vi "PDW gen.vi"() -> ()   [LabVIEW 2021]
uses:
  emitter params.ctl
  pdw.ctl
  <vilib>/numeric/Random Number (Range) DBL.vi
  <vilib>/numeric/Random Number (Range) U64.vi
  <vilib>/numeric/sub_Random U32.vi
panel:
  out "lfm lost":bool
  in  "Tab Control":T1(tab)
  in  "end time (sec)":dbl=50.0
  in  "start time (sec)":dbl format="%#_13g"
  in  "Fs":i32=200000000 format="%.0p"
  in  "tdms output file path":path=path "C:/Users/NI/Documents/chaim/chaim__Tx/data/pulses.tdms"
  in  "center frequency (Hz)":dbl=2000000000.0 format="%#_13p"
  in  "amp range":cluster{dbl, dbl}(slide)={-21.121351766513058, -25.88325652841782} scale=0.0..-50.0 scale format="%#_g dB"
  in  "span range":cluster{dbl, dbl}(slide)={1634128.9560392164, 2964508.639841233} scale=1000000.0..30000000.0 scale format="%#_6p Hz"
  in  "hop rate range":cluster{dbl, dbl}(slide)={2.0915680786684536, 3.1385684721559217} scale=1.0..3000.0 scale format="%#_6p"
  in  "D.C range":cluster{dbl, dbl}(slide)={0.5407066052227343, 0.5038402457757296} scale=0.0..1.0
  in  "f band range":cluster{dbl, dbl}(slide)={-77296466.97388633, 78525345.62211981} scale=-80000000.0..80000000.0 scale format="%#_6p Hz"
  in  "CW":bool=TRUE
  in  "LFM":bool=TRUE
  in  "BPSK":bool=TRUE
  in  "QPSK":bool=TRUE
  in  "num of frequncyes":cluster{i32, i32}(slide)={2, 1} scale=1.0..300.0
  in  "num of hoopers":i32(slide)=10 scale=0.0..16.0
  in  "modulation depth":cluster{dbl, dbl}(slide)={67532.40039072247, 205475.5312375231} scale=10000.0..3000000.0 scale format="%#_6p Hz"
  in  "user bulid emmiters":T2[](array[typedef]) {"mod depth" format="%.0p"; "f set" format="%#_6p"}
  out "PDW":T3={"PW"=44197525, "frequency shift"=-0.34743934348748695, "amp"=0.06598663330078125, "mode type"=4, "mode depth"=1109, "mode filter"=0}
  out "saturation":bool
  out "num of pulses":i32=1261
  # "available modulations:"
  # "mode type:\n0-CW\n3-LFM\n4-BPSK\n5-QPSK"
  # "mode type:\n0-CW\n3-LFM\n4-BPSK\n5-QPSK"
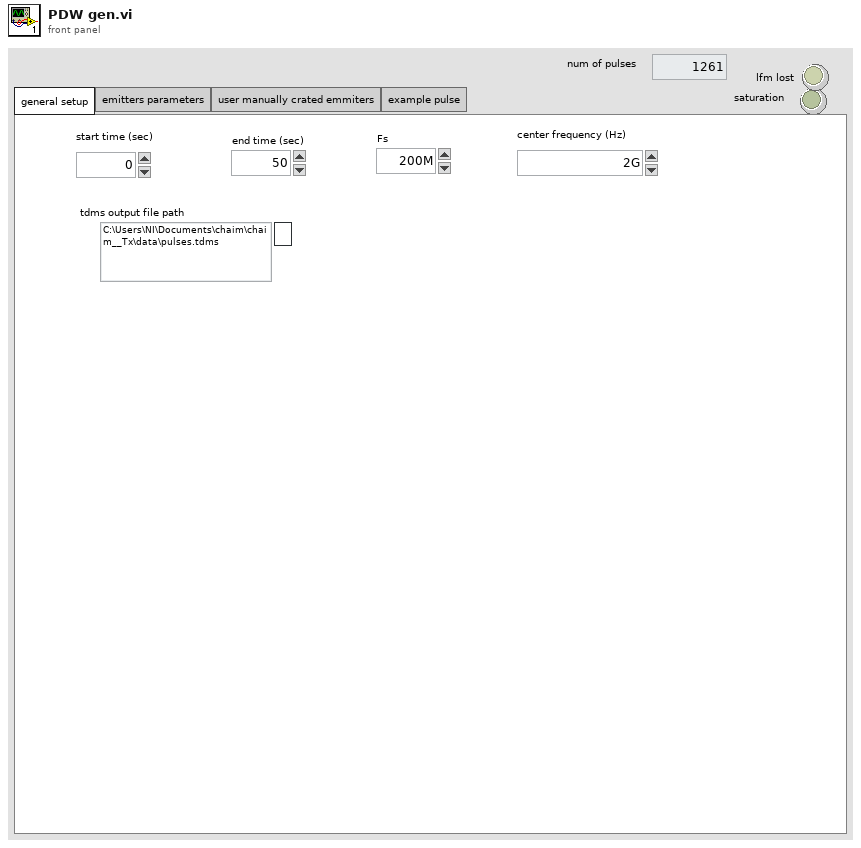
[diagram p1: front panel]
types:
  T1 = enum32{"general setup", "emitters parameters", "user manually crated emmiters", "example pulse"}
  T2 = typedef "emitter params.ctl" = cluster{"f set":dbl[], "hop rate (Hz)":dbl, "d.c.":dbl, "amp (dB)":dbl, "mod type":u8, "mod depth":dbl}
  T3 = typedef "pdw.ctl" = cluster{"PW":u32, "frequency shift":fxp<+/-,48,0>, "amp":fxp<+/-,18,1>, "mode type":u8, "mode depth":u32, "mode filter":u8}
  T4 = enum16{"open", "open or create", "create or replace", "create", "open (read-only)"}
  T5 = cluster{"start time":dbl, "Numeric":dbl, dbl, "amp (dB)":dbl, "mod type":u8, "mod file 2":u8, "mod depth":dbl, "pulse filter":u16, "mod filter 2":u16}[]
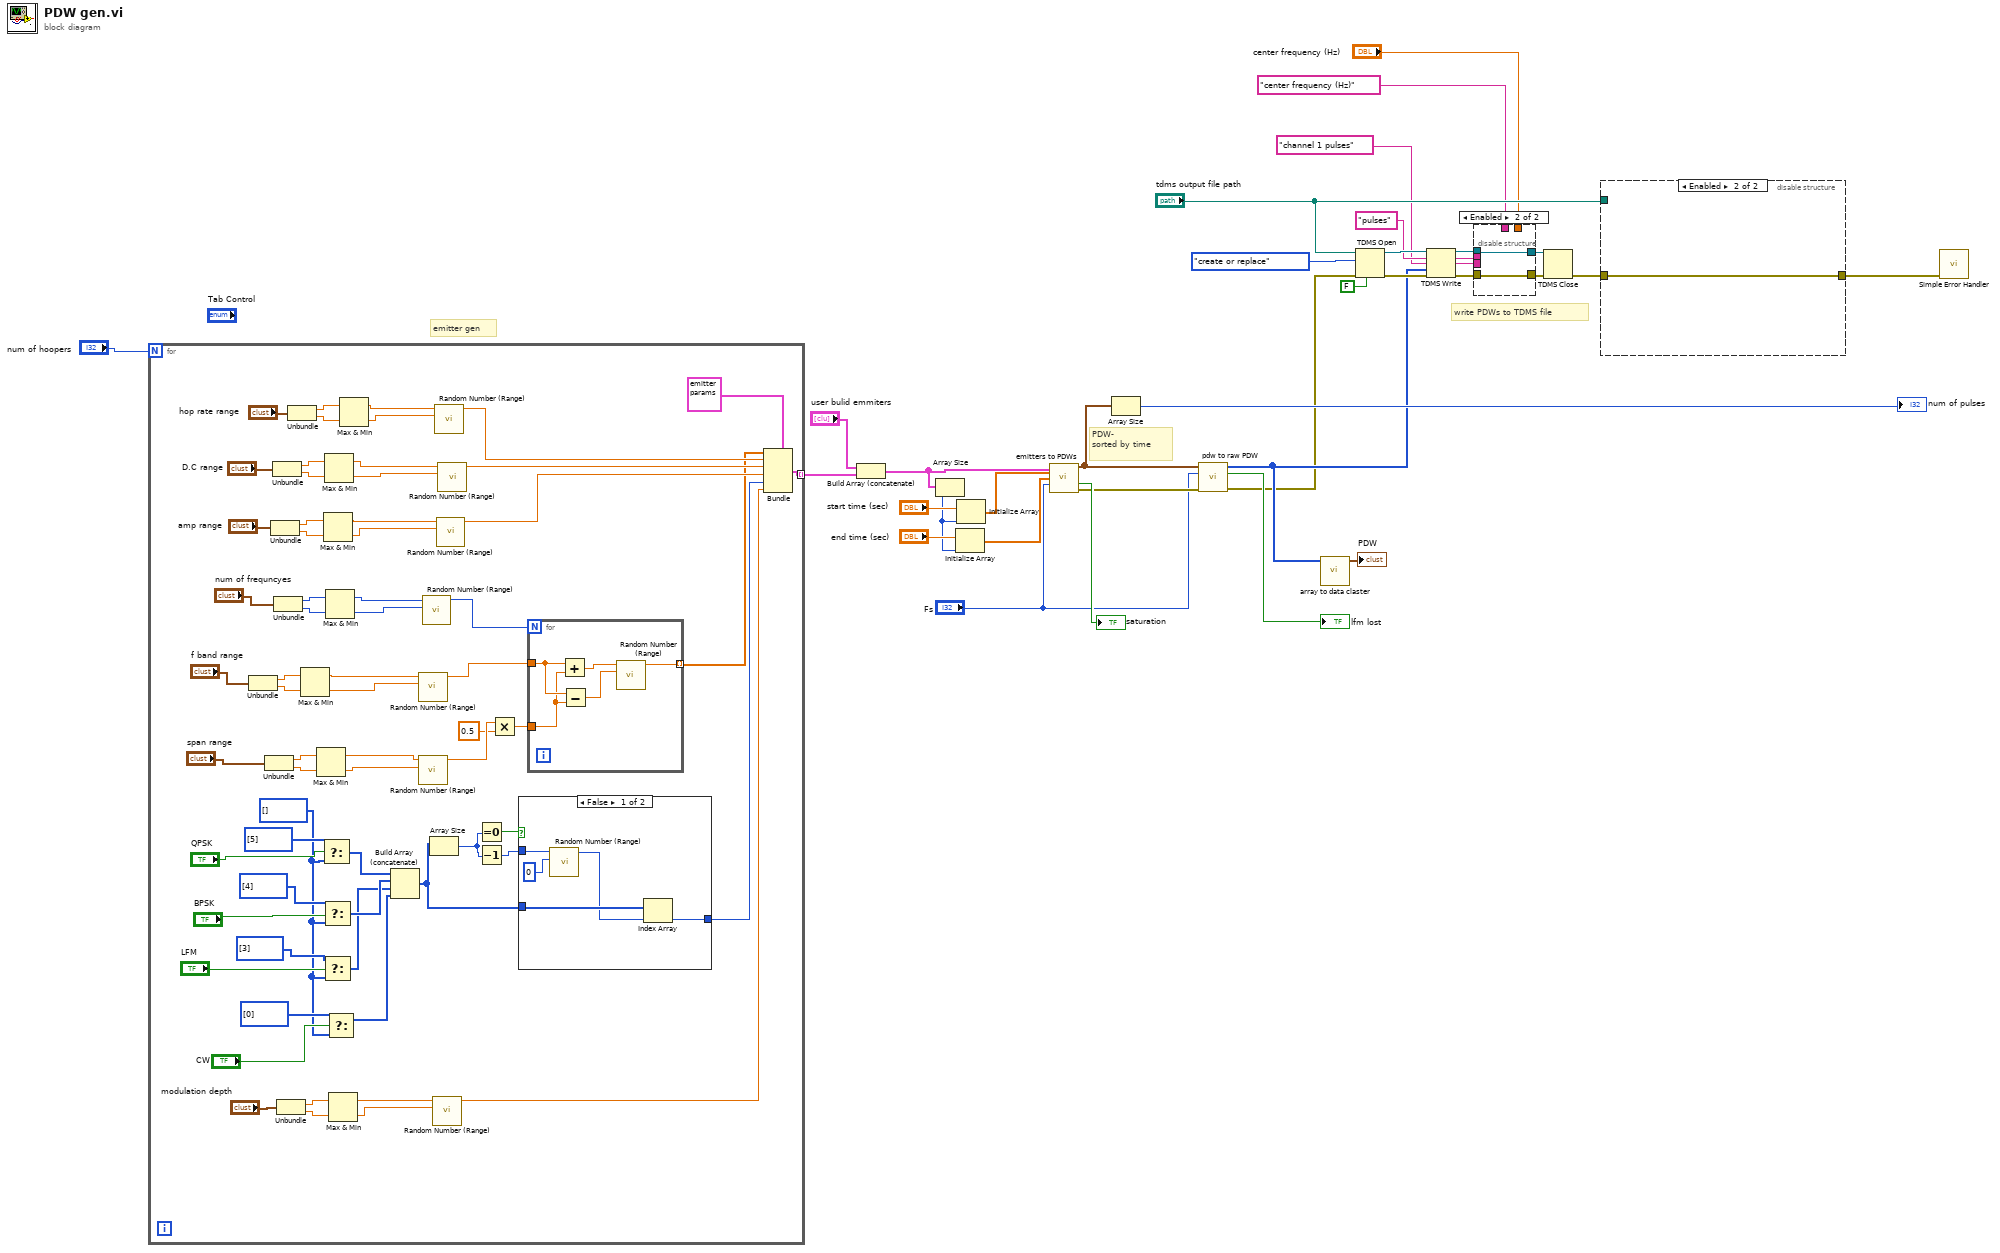
[diagram p0: block diagram]
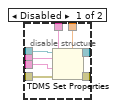
[diagram p2: hidden frame]
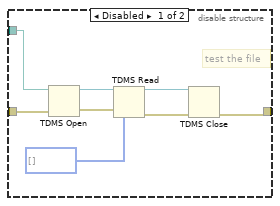
[diagram p3: hidden frame]
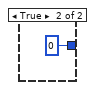
[diagram p4: hidden frame]
diagram:
  # "write PDWs to TDMS file"
  # "PDW- \nsorted by time"
  # "emitter gen"
  n1 = for {
    N: "num of hoopers" -> [_]
    tunnel: [w91] -> w34 mode=indexing
    w36 = u8[] []
    n2 = Unbundle("f band range") -> (w69:dbl, w68:dbl)
    n3 = Unbundle("span range") -> (w63:dbl, w64:dbl)
    n4 = Unbundle("amp range") -> (w87:dbl, w86:dbl)
    n5 = Unbundle("D.C range") -> (w83:dbl, w84:dbl)
    n6 = Unbundle("num of frequncyes") -> (w73:i32, w74:i32)
    n7 = Unbundle("modulation depth") -> (w59:dbl, w58:dbl)
    n8 = Unbundle("hop rate range") -> (w79:dbl, w78:dbl)
    n9 = Max & Min(x=w69, y=w68) -> (max(x,y)=w66:dbl, min(x,y)=w65:dbl)
    n10 = Max & Min(x=w63, y=w64) -> (max(x,y)=w62:dbl, min(x,y)=w61:dbl)
    n11 = Select(t=u8[] [5], s="QPSK", f=w36) -> (s? t:f=w50:u8[])
    n12 = Max & Min(x=w87, y=w86) -> (max(x,y)=w89:dbl, min(x,y)=w88:dbl)
    n13 = Select(t=u8[] [4], s="BPSK", f=w36) -> (s? t:f=w49:u8[])
    n14 = Select(t=u8[] [3], s="LFM", f=w36) -> (s? t:f=w48:u8[])
    n15 = Max & Min(x=w83, y=w84) -> (max(x,y)=w82:dbl, min(x,y)=w81:dbl)
    n16 = Max & Min(x=w73, y=w74) -> (max(x,y)=w71:i32, min(x,y)=w70:i32)
    n17 = Select(t=u8[] [0], s="CW", f=w36) -> (s? t:f=w47:u8[])
    n18 = Max & Min(x=w59, y=w58) -> (max(x,y)=w56:dbl, min(x,y)=w55:dbl)
    n19 = Max & Min(x=w79, y=w78) -> (max(x,y)=w76:dbl, min(x,y)=w75:dbl)
    n20 = Build Array (concatenate)(w50, w49, w48, w47) -> (w46:u8[])
    n21 = call-poly <vilib>:"Random Number (Range).vi"("lower bound (0)"=w65, "upper bound (100)"=w66) -> ("number"=w94:dbl)  [unwired: 9 in]
    n22 = call-poly <vilib>:"Random Number (Range).vi"("lower bound (0)"=w61, "upper bound (100)"=w62) -> ("number"=w96:dbl)  [unwired: 9 in]
    n23 = call-poly <vilib>:"Random Number (Range).vi"("lower bound (0)"=w70, "upper bound (100)"=w71) -> ("number"=w90:u64)  [unwired: 9 in]
    n24 = Array Size(array=w46) -> (size(s)=w42:i32)
    n25 = call-poly <vilib>:"Random Number (Range).vi"("lower bound (0)"=w55, "upper bound (100)"=w56) -> ("number"=w43:dbl)  [unwired: 9 in]
    n26 = call-poly <vilib>:"Random Number (Range).vi"("lower bound (0)"=w75, "upper bound (100)"=w76) -> ("number"=w99:dbl)  [unwired: 9 in]
    n27 = call-poly <vilib>:"Random Number (Range).vi"("lower bound (0)"=w88, "upper bound (100)"=w89) -> ("number"=w97:dbl)  [unwired: 9 in]
    n28 = call-poly <vilib>:"Random Number (Range).vi"("lower bound (0)"=w81, "upper bound (100)"=w82) -> ("number"=w98:dbl)  [unwired: 9 in]
    n29 = Equal To 0?(x=w42) -> (x = 0?=w44:bool)
    n30 = Decrement(x=w42) -> (x-1=w41:i32)
    n31 = Multiply(x=w96, y=0.5) -> (x*y=w93:dbl)
    n32 = case shown="False" w44 {
      tunnel: w46 -> [w104 _]
      tunnel: [w102 u8 0 ("unsigned 8bit integer")] -> w45
      tunnel: w41 -> [w101 _]
      frame False {
        n33 = call-poly <vilib>:"Random Number (Range).vi"("lower bound (0)"=u64 0, "upper bound (100)"=w101) -> ("number"=w103:u64)  [unwired: 9 in]
        n34 = Index Array(array=w104, index=w103) -> (element=w102:u8)
      }
      frame True {
      }
    }
    n35 = for {
      N: w90 -> [_]
      tunnel: w94 -> [w111]
      tunnel: w93 -> [w110]
      tunnel: [w107] -> w92 mode=indexing
      n36 = Add(x=w111, y=w110) -> (x+y=w108:dbl)
      n37 = Subtract(x=w111, y=w110) -> (x-y=w109:dbl)
      n38 = call-poly <vilib>:"Random Number (Range).vi"("lower bound (0)"=w109, "upper bound (100)"=w108) -> ("number"=w107:dbl)  [unwired: 9 in]
    }
    n39 = Bundle(cluster=T2 {"f set"=[1000000.0], "hop rate (Hz)"=300000.0, "d.c."=0.0, "amp (dB)"=-20.0, "mod type"=0, "mod depth"=0.0} ("Cluster"), "f set"=w92, "hop rate (Hz)"=w99, "d.c."=w98, "amp (dB)"=w97, "mod type"=w45, "mod depth"=w43) -> (w91:T2)
  }
  n40 = Build Array (concatenate)("user bulid emmiters", w34) -> (w24:T2[])
  n41 = Array Size(array=w24) -> (size(s)=w21:i32)
  n42 = Initialize Array("end time (sec)", w21) -> (w19:dbl[])
  n43 = Initialize Array("start time (sec)", w21) -> (w20:dbl[])
  n44 = call "emitters to PDWs.vi"("emmiter"=w24, "start time"=w20, "end time"=w19, "fs [Hz]"="Fs") -> ("sorted array"=w26:T5, "may saturate"=→"saturation":bool, "erorr out"=w13:errorcluster)  [unwired: 9 in]
  n45 = Array Size(array=w26) -> (size(s)=→"num of pulses":i32)
  n46 = call "pdw to raw PDW.vi"("erorr in"=w13, "Fs"="Fs", "PDW"=w26) -> ("erorr out"=w12:errorcluster, "lfm lost"=→"lfm lost":bool, "Array"=w16:u64[])  [unwired: 6 in]
  n47 = call "array to data claster.vi"("Array"=w16) -> ("Cluster"=→"PDW":T3)  [unwired: 10 in]
  n48 = TDMS Open(6:FALSE ("enable asynchronous? (T)"), 8:w12, 10:T4."create or replace" ("operation (0:open)"), 11:"tdms output file path") -> (0:w33:errorcluster, 3:w30:refnum<k34>)  [unwired: 3 in]
  n49 = TDMS Write(0:w30, 5:"pulses" ("group name in (Untitled)"), 7:"channel 1 pulses", 9:w16, 11:w33) -> (4:w8:refnum<k34>, 6:w4:string, 8:w3:string, 15:w7:errorcluster)  [unwired: 1 in]
  n50 = disable-structure shown="Enabled" {
    disable-tunnel: w8 -> [w119 w121]
    disable-tunnel: w7 -> [w118 w120]
    disable-tunnel: [w117 w121] -> w6
    disable-tunnel: [w116 w120] -> w5
    disable-tunnel: w4 -> [w115 _]
    disable-tunnel: w3 -> [w114 _]
    disable-tunnel: "center frequency (Hz)" -> [w113 _]
    disable-tunnel: "center frequency (Hz)" -> [w112 _]
    frame Disabled {
      n51 = TDMS Set Properties(5:w113, 7:w112, 8:w118, 9:w114, 10:w115, 11:w119) -> (0:w116:errorcluster, 3:w117:refnum<k34>)  [unwired: 2 out]
    }
    frame Enabled {
    }
  }
  n52 = TDMS Close(8:w5, 11:w6) -> (0:w27:errorcluster)  [unwired: 1 out]
  n53 = disable-structure "Diagram Disable Structure" shown="Enabled" {
    disable-tunnel: "tdms output file path" -> [w126 _]
    disable-tunnel: w27 -> [w123 w130]
    disable-tunnel: [w122 w130] -> w18
    frame Disabled {
      # "test the file"
      n54 = TDMS Open(8:w123, 11:w126) -> (0:w128:errorcluster, 3:w125:refnum<k34>)  [unwired: 5 in]
      n55 = TDMS Read(0:w125, 11:w128, 12:u64[] [] ("Data")) -> (4:w124:refnum<k34>, 15:w127:errorcluster)  [unwired: 5 in, 4 out]
      n56 = TDMS Close(8:w127, 11:w124) -> (0:w122:errorcluster)  [unwired: 1 out]
    }
    frame Enabled {
    }
  }
  n57 = call <vilib>:"Simple Error Handler.vi"("error in (no error)"=w18) -> ()  [unwired: 4 in, 5 out]
